vi "Vision Research Phantom Series PhFile PhDuplicateCine.vi"(0 "hCSrc [in]":i32, 5 "Error In (no error)":errorcluster) -> (14 "hCSrc [out]":i32, 15 "phCDest [out]":i32, 19 "Error Out":errorcluster)   [LabVIEW 2013, in "VRI.lvlib"]
doc: "PhDuplicateCine\nHRESULT PhDuplicateCine(PCINEHANDLE phCDest, CINEHANDLE hCSrc);\n\nParameters\nphCDest [out]\n Pointer or to store a new cine handle created by duplicating hCSrc.\nhCSrc [in]\n Source cine to be duplicated.\n\nReturn Value\nThe function returns ERR_Ok in case of success or an error code, otherwise. To get the text of the error message call PhGetErrorMessage.\n\nRemarks\nIt creates a duplicate of the input cine. It cannot be used for live cines.\nUse this function when needing to run in parallel different operations for the same cine (e.g. reading images for display and reading images for saving to file) if cine parameters have changed from the moment the cine was created. Since some parameters are stored in internal buffers only, a PhNewCineFromCamera or PhNewCineFromFile call will also create a new cine, but it will not be aware of the parameters previously changed. This can happen especially for file cines where an image processing parameter change is stored only in internal buffers and written to file just when the cine is saved.\nCall PhDestroyCine after finishing working with the duplicate cine.\n\nRequired Header\n PhFile.h"
uses:
  VRI.lvlib
  Phantom DLLs/PhFile.Dll
panel:
  # "For instructions on the use of this VI, press Ctrl+H to display the help window and move the mouse over the icon, controls, and indicators"
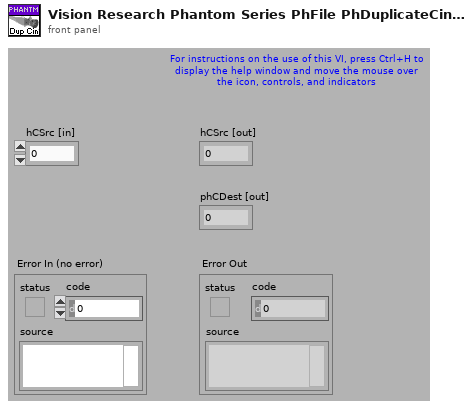
[diagram p1: front panel]
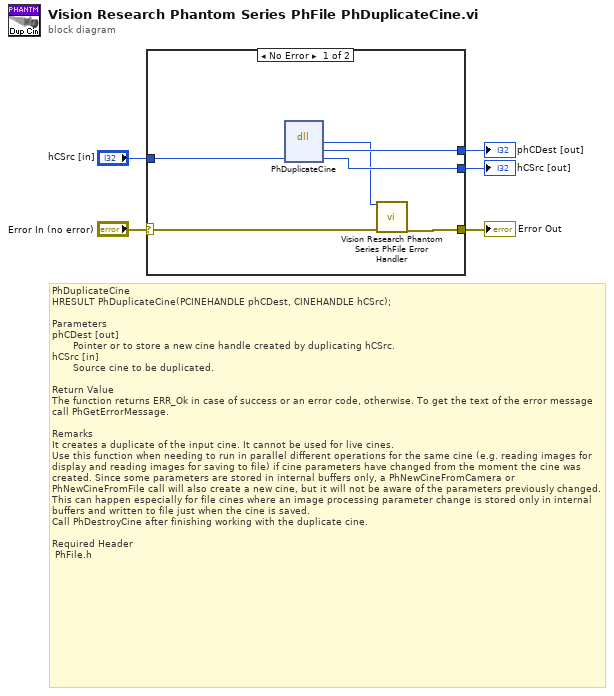
[diagram p0: block diagram]
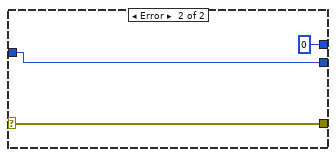
[diagram p2: hidden frame]
diagram:
  # "PhDuplicateCine\nHRESULT PhDuplicateCine(PCINEHANDLE phCDest, CINEHANDLE hCSrc);\n\nParameters\nphCDest [out]\n\t      Pointer or to store a new cine handle created by duplicating hCSrc.\nhCSrc [in]\n\t      Source cine to be duplicated.\n\nReturn Value\nThe function returns ERR_Ok in case of success or an error code, otherwise. To get the text of the error message call PhGetErrorMessage.\n\nRemarks\nIt creates a duplicate of the input cine. It cannot be used for live cines.\nUse this function when needing to run in parallel different operations for the same cine (e.g. reading images for display and reading images for saving to file) if cine parameters have changed from the moment the cine was created. Since some parameters are stored in internal buffers only, a PhNewCineFromCamera or PhNewCineFromFile call will also create a new cine, but it will not be aware of the parameters previously changed. This can happen especially for file cines where an image processing parameter change is stored only in internal buffers and written to file just when the cine is saved.\nCall PhDestroyCine after finishing working with the duplicate cine.\n\nRequired Header\n\tPhFile.h"
  n1 = case shown="No Error" "Error In (no error)" {
    selector: "Error In (no error)" -> [w11 w14]
    tunnel: [w10 w14] -> w4
    tunnel: "hCSrc [in]" -> [w9 w13]
    tunnel: [w8 0 ("phCDest")] -> w2
    tunnel: [w7 w13] -> w1
    frame No Error {
      n2 = dll-call lib="C:/Projects/SDK/64-bit/Vision Research Phantom Series Labview Driver/Phantom DLLs/PhFile.dll" fn="PhDuplicateCine"("hCSrc"=w9) -> ("HRESULT"=w6:i32, "phCDest"=w8:i32, "hCSrc"=w7:i32)  [unwired: 3 in, 3 out]
      n3 = call "Vision Research Phantom Series PhFile Error Handler.vi"("Error Code (0)"=w6, "Error In (no error)"=w11) -> ("Error Out"=w10:errorcluster)  [unwired: 17 out]
    }
    frame Error {
    }
  }
  "Error Out" <- w4
  "phCDest [out]" <- w2
  "hCSrc [out]" <- w1
